vi "Gray_conv.vi"(4 "D":bool, 5 "C":bool, 6 "B":bool, 7 "A":bool) -> (0 "A0":bool, 1 "A1":bool, 2 "A2":bool, 3 "A3":bool)   [LabVIEW 2016]
doc: "Este Instrumento Vitual hace una conversión de Binario a Código Gray.\nLa Entrada A es la mas significativa y la D la menos significativa."
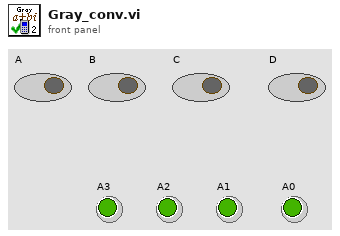
[diagram p1: front panel]
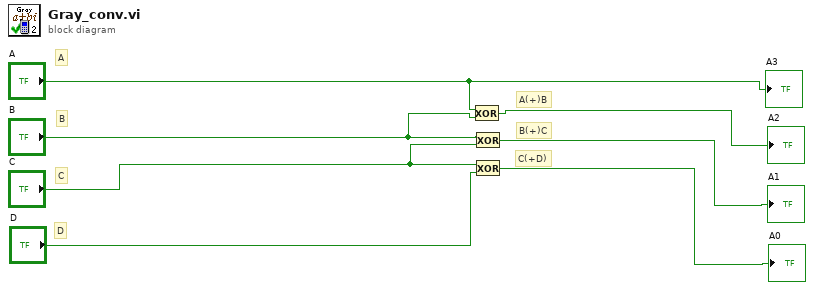
[diagram p0: block diagram]
diagram:
  # "C(+D)"
  # "B(+)C"
  # "A(+)B"
  # "D"
  # "C"
  # "B"
  # "A"
  n1 = Exclusive Or(1:"B", 2:"A") -> (0:→"A2":bool)
  n2 = Exclusive Or(1:"C", 2:"B") -> (0:→"A1":bool)
  n3 = Exclusive Or(1:"D", 2:"C") -> (0:→"A0":bool)
  "A3" <- "A"
